vi "Intake_Execute.vi"() -> ()   [LabVIEW 2019]
uses:
  <vilib>/Rock Robotics/WPI/ThirdParty/REV Robotics/SPARK MAX/Typedef/Spark MAX Control Type.ctl
  <vilib>/Rock Robotics/WPI/Solenoid/WPI_SolenoidValue.ctl
  Intake_Cluster.ctl
  Intake_States.ctl
  Globals/Intake_Globals.vi
  Globals/Solenoid Globals.vi
  <vilib>/Rock Robotics/WPI/Solenoid/WPI_SolenoidSetEnum.vi
panel:
  in  "Intake_Speed":dbl=0.875
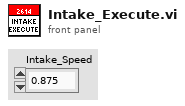
[diagram p1: front panel]
types:
  T1 = typedef "WPI_MotorControlDeviceRef.ctl" = cluster{"DeviceStatus":errorcluster, "Type":T2, "PWM":cluster{"PWM Channel":T3, "DeadBand":T4}, "CAN":cluster{"Device Number":u8, "SetOutput VI Ref":variant, "GetOutput VI Ref":variant, "Enable VI Ref":variant, "Disable VI Ref":variant, "Data":variant}, "Invert":bool, "DIO PWM":cluster{"PWM \"Enable\" Channel":T3, "DIOChannel":T5, "PWM Rate":dbl}}
  T2 = typedef "WPI_MotorControlType.ctl" = enum16{"PWM", "CAN", "DIO PWM"}
  T3 = typedef "FPGA_DIOPWMChannel.ctl" = enum8{"PWM 0", "PWM 1", "PWM 2", "PWM 3", "PWM 4", "PWM 5", "PWM 6", "PWM 7", "PWM 8", "PWM 9", "PWM MXP 0", "PWM MXP 1", "PWM MXP 2", "PWM MXP 3", "PWM MXP 4", "PWM MXP 5", "PWM MXP 6", "PWM MXP 7", "PWM MXP 8", "PWM MXP 9", "Invalid"}
  T4 = typedef "WPI_PWMDeadband.ctl" = cluster{"Name":string, "maxPositivePwm":i32, "minPositivePwm":i32, "centerPwm":i32, "maxNegativePwm":i32, "minNegativePwm":i32, "angularRange":u16}
  T5 = typedef "FPGA_DIOChannel.ctl" = enum8{"DIO 0", "DIO 1", "DIO 2", "DIO 3", "DIO 4", "DIO 5", "DIO 6", "DIO 7", "DIO 8", "DIO 9", "DIO MXP 0", "DIO MXP 1", "DIO MXP 2", "DIO MXP 3", "DIO MXP 4", "DIO MXP 5", "DIO MXP 6", "DIO MXP 7", "DIO MXP 8", "DIO MXP 9", "DIO MXP 10", "DIO MXP 11", "DIO MXP 12", "DIO MXP 13", "DIO MXP 14", "DIO MXP 15", "SPI Port CS1", "SPI Port CS2", "SPI Port CS3", "SPI Port MISO", "SPI Port MOSI", "Invalid"}
  T6 = typedef "WPI_SolenoidDevRef.ctl" = cluster{"DevStatus":errorcluster, "Pneumatics Control Module":u8, "Forward Solenoid Channel":T7, "Reverse Solenoid Channel":T7}
  T7 = typedef "WPI_SolenoidChannel.ctl" = enum8{"Solenoid 0", "Solenoid 1", "Solenoid 2", "Solenoid 3", "Solenoid 4", "Solenoid 5", "Solenoid 6", "Solenoid 7", "Invalid"}
  T8 = typedef "WPI_SolenoidValue.ctl" = enum16{"Off", "On", "Forward", "Reverse"}
  T9 = typedef "Intake_Cluster.ctl" = cluster{"Control_State":T10, "Intake_On":bool, "Intake_Extended":bool, "Intake_Throttle":dbl, "Auto_Notifier":refnum<notifier>, "Parameter_1":dbl, "Parameter_2":dbl, "Step":dbl, "Outtake":bool}
  T10 = typedef "Intake_States.ctl" = enum16{"Manual_Control", "Compliant_Intake"}
  T11 = typedef "Spark MAX Control Type.ctl" = enum16{"Percent VBus", "Voltage", "Velocity", "Position", "Smart Motion", "Current", "Smart Velocity"}
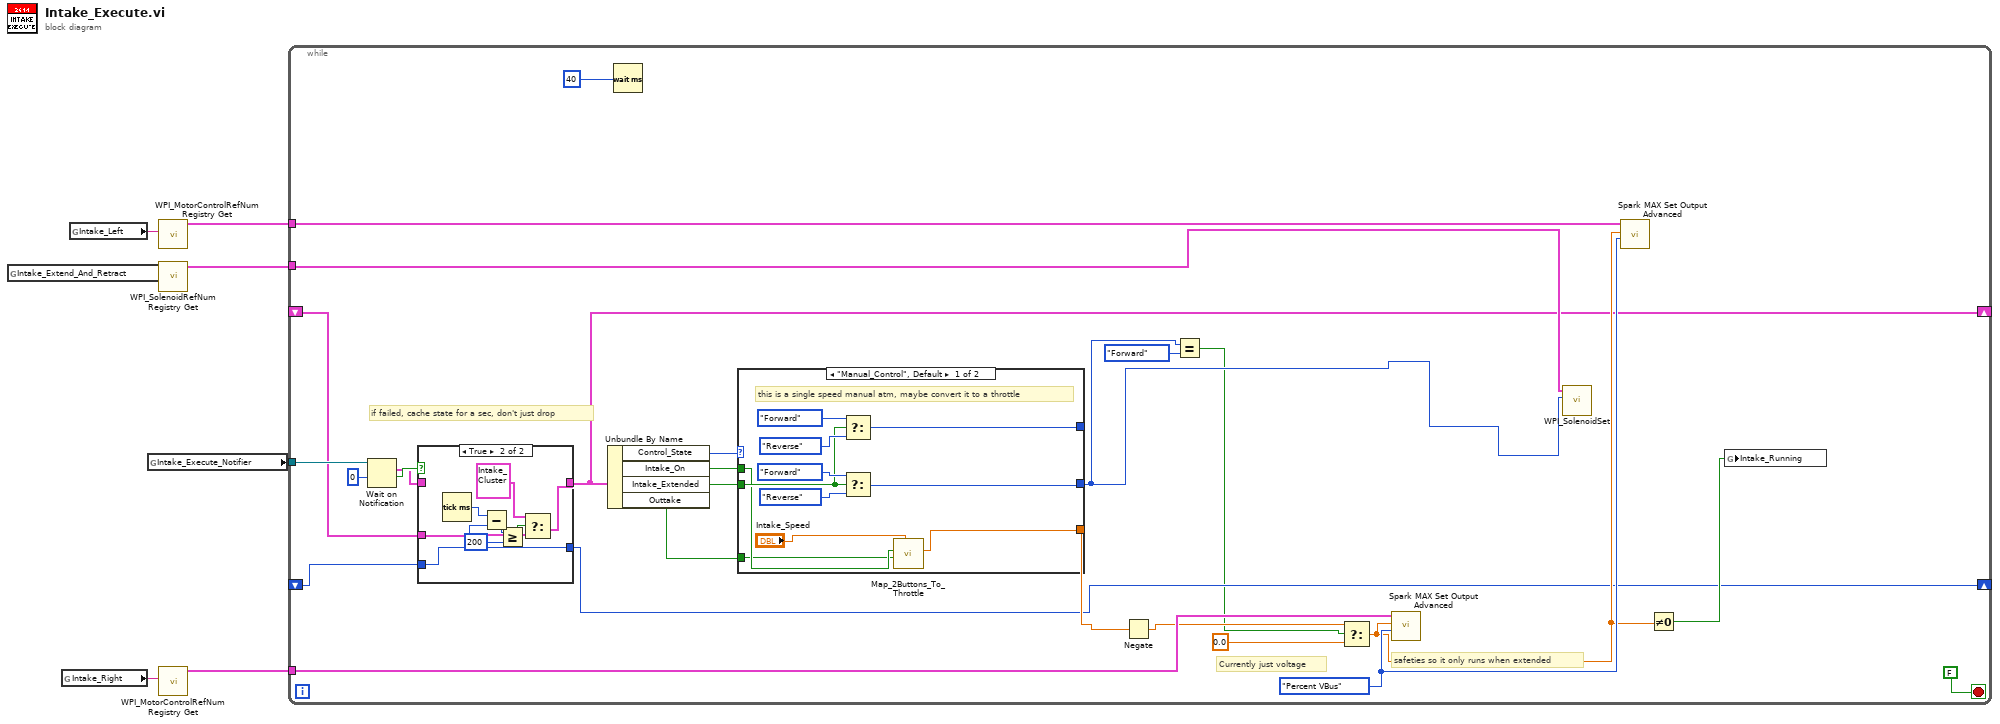
[diagram p0: block diagram]
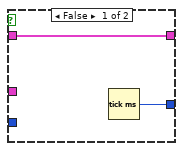
[diagram p2: hidden frame]
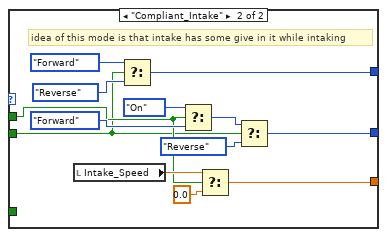
[diagram p3: hidden frame]
diagram:
  n1 = global read "Solenoid Globals.vi" "Intake_Extend_And_Retract"() -> (w2:string)
  n2 = global read "Intake_Globals.vi" "Intake_Right"() -> (w6:string)
  n3 = global read "Intake_Globals.vi" "Intake_Left"() -> (w5:string)
  n4 = global read "Intake_Globals.vi" "Intake_Execute_Notifier"() -> (w7:refnum<notifier>)
  n5 = call <vilib>:"WPI_MotorControlRefNum Registry Get.vi"("refnum name"=w5) -> ("MotorControlDevRef"=w4:T1)  [unwired: 9 in, 1 out]
  n6 = call <vilib>:"WPI_SolenoidRefNum Registry Get.vi"("refnum name"=w2) -> ("SolenoidDevRef"=w1:T6)  [unwired: 9 in, 1 out]
  n7 = call <vilib>:"WPI_MotorControlRefNum Registry Get.vi"("refnum name"=w6) -> ("MotorControlDevRef"=w3:T1)  [unwired: 9 in, 1 out]
  n8 = while {
    tunnel: w7 -> [w32]
    tunnel: w4 -> [w28]
    tunnel: w3 -> [w27]
    tunnel: w1 -> [w25]
    shift-right: [w12] -> _
    shift-left: _ -> [w11]
    shift-right: [w10] -> _
    shift-left: _ -> [w9]
    stop <- FALSE stop-if-true
    w26 = Spark_MAX_Control_Type."Percent VBus" ("Control Mode")
    # "if failed, cache state for a sec, don't just drop"
    # "Currently just voltage"
    # "safeties so it only runs when extended"
    n9 = Wait on Notification(notifier=w32, timeout in ms (-1)=0) -> (notification=w13:T9, timed out?=w15:bool)  [unwired: 2 in, 2 out]
    n10 = case shown="True" w15 {
      tunnel: w13 -> [w35 _]
      tunnel: [w35 w43] -> w12
      tunnel: w11 -> [_ w42]
      tunnel: [w34 w40] -> w10
      tunnel: w9 -> [_ w40]
      frame False {
        n11 = Tick Count (ms)() -> (millisecond timer value=w34:u32)
      }
      frame True {
        n12 = Tick Count (ms)() -> (millisecond timer value=w41:u32)
        n13 = Subtract(x=w41, y=w40) -> (x-y=w38:u32)
        n14 = Greater Or Equal?(x=w38, y=u32 200) -> (x >= y?=w39:bool)
        n15 = Select(t=T9 {"Control_State"=enum."Manual_Control", "Intake_On"=FALSE, "Intake_Extended"=FALSE, "Intake_Throttle"=0.0, "Auto_Notifier"=refnum, "Parameter_1"=0.0, "Parameter_2"=0.0, "Step"=0.0, "Outtake"=FALSE}, s=w39, f=w42) -> (s? t:f=w43:T9)
      }
    }
    n16 = Unbundle By Name(w12) -> ("Control_State"=w31:T10, "Intake_On"=w30:bool, "Intake_Extended"=w20:bool, "Outtake"=w22:bool)
    n17 = Wait (ms)(milliseconds to wait=u32 40) -> ()  [unwired: 1 out]
    n18 = case shown="\"Manual_Control\", Default" w31 {
      tunnel: w20 -> [w49 w57]
      tunnel: [w52 w64] -> w21
      tunnel: w30 -> [w47 w60]
      tunnel: [w44 w55] -> w19
      tunnel: [w48 w56] -> _
      tunnel: w22 -> [w46 _]
      frame "Manual_Control", Default {
        # "this is a single speed manual atm, maybe convert it to a throttle"
        n19 = Select(t=WPI_SolenoidValue."Forward" ("Value"), s=w49, f=WPI_SolenoidValue."Reverse" ("Value")) -> (s? t:f=w48:T8)
        n20 = Select(t=WPI_SolenoidValue."Forward" ("Value"), s=w49, f=WPI_SolenoidValue."Reverse" ("Value")) -> (s? t:f=w52:T8)
        n21 = call "Map_2Buttons_To_Throttle.vi"("Power"="Intake_Speed", "Down"=w46, "Up"=w47) -> ("Throttle"=w44:dbl)  [unwired: 8 in]
      }
      frame "Compliant_Intake" {
        # "idea of this mode is that intake has some give in it while intaking"
        n22 = local read "Intake_Speed"() -> (w65:dbl)
        n23 = Select(t=WPI_SolenoidValue."Forward" ("Value"), s=w57, f=WPI_SolenoidValue."Reverse" ("Value")) -> (s? t:f=w56:T8)
        n24 = Select(t=WPI_SolenoidValue."On" ("Value"), s=w60, f=WPI_SolenoidValue."Forward" ("Value")) -> (s? t:f=w63:T8)
        n25 = Select(t=w65, s=w60, f=0.0) -> (s? t:f=w55:dbl)
        n26 = Select(t=w63, s=w57, f=WPI_SolenoidValue."Reverse" ("Value")) -> (s? t:f=w64:T8)
      }
    }
    n27 = Negate(x=w19) -> (-x=w18:dbl)
    n28 = Equal?(x=w21, y=WPI_SolenoidValue."Forward") -> (x = y?=w8:bool)
    n29 = Select(t=w18, s=w8, f=0.0) -> (s? t:f=w17:dbl)
    n30 = call <vilib>:"Spark MAX Set Output Advanced.vi"("Control Mode"=w26, "Setpoint"=w17, "MotorControlDevRef"=w27) -> ()  [unwired: 7 in, 2 out]
    n31 = call-poly <vilib>:"WPI_SolenoidSet.vi"("Value"=w21, "SolenoidDevRef"=w25) -> ()  [unwired: 8 in, 2 out]
    n32 = call <vilib>:"Spark MAX Set Output Advanced.vi"("Control Mode"=w26, "Setpoint"=w17, "MotorControlDevRef"=w28) -> ()  [unwired: 7 in, 2 out]
    n33 = Not Equal To 0?(x=w17) -> (x != 0?=w16:bool)
    n34 = global write "Intake_Globals.vi" "Intake_Running"(w16) -> ()
  }
